vi "Connection Test.vi"() -> ()   [LabVIEW 2015]
uses:
  <vilib>/Rock Robotics/SystemInterfaces/spilib/spi_bus.ctl
  <vilib>/Platform/TimedLoop/XDataNode/timing_clust.ctl
  <vilib>/Platform/TimedLoop/XDataNode/nitl_modes.ctl
  <vilib>/Platform/TimedLoop/XDataNode/wakeup.ctl
  <vilib>/Rock Robotics/SystemInterfaces/i2clib/i2c_bus.ctl
  navX Library v3/navX Registry Cache/_TypeDefs/DeviceRegistryTypeDef.ctl
  navX Library v3/navX/navX.lvclass/navX.ctl
  navX Library v3/navX - Interface/navX - Interface.lvclass/navX - Interface.ctl
  navX Library v3/navX/_Open/OpenSPI.vi
  navX Library v3/navX - Interface/Notifications/Send Notification.vi
  <vilib>/platform/TimedLoop/XDataNode/XDataNode.xnode
  navX Library v3/navX - Interface/navX - Interface.lvclass
  navX Library v3/navX/navX.lvclass
  <vilib>/Platform/TimedLoop/XDataNode/XDNodeRunTimeDep.lvlib
  navX Library v3/navX Registry Cache/navX Registry Cache.lvclass
panel:
  out "Timestamp":u32
  in  "Update Rate (4Hz-100Hz)":u8=4 min=4 max=100 step=1
  in  "Update Button":bool
  out "YPRHfH":T1
  in  "stop":bool
  out "Iteration Duration":i64
  out "Finished Late? [i-1]":bool
  out "Registry":u8[][](array[numeric])
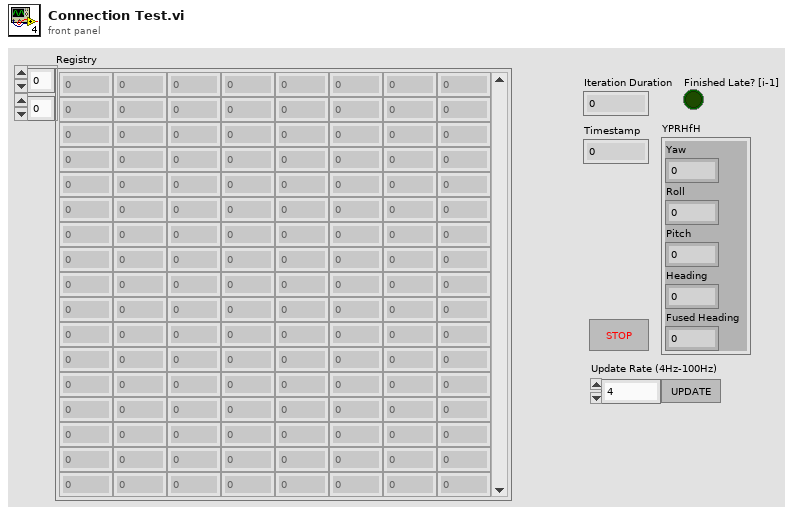
[diagram p1: front panel]
types:
  T1 = cluster{"Yaw":dbl, "Roll":dbl, "Pitch":dbl, "Heading":dbl, "Fused Heading":dbl}
  T2 = typedef "i2c_bus.ctl" = enum16{"I2C On-Board", "I2C MXP", "Invalid"}
  T3 = typedef "spi_bus.ctl" = enum16{"SPI On-Board, CS0", "SPI On-Board, CS1", "SPI On-Board, CS2", "SPI On-Board, CS3", "SPI MXP", "Invalid"}
  T4 = typedef "XDNodeRunTimeDep.lvlib/timing_clust.ctl" = cluster{"Expected End [f-1]":u64, "Actual End [f-1]":u64, "Finished Late? [f-1]":bool, "Expected End [i-1]":u64, "Actual End [i-1]":u64, "Finished Late? [i-1]":bool, "Expected Start [i]":u64, "Actual Start [i]":u64, "Expected Start [f]":u64, "Actual Start [f]":u64, "Source Name":string, "Structure Name":string, "Period":i64, "Deadline":i64, "Offset":i64, "Start":i64, "Priority":i32, "Timeout":i32, "Mode":T5, "Wakeup Reason":T6, "Error":errorcluster, "Source Type":string, "Secondary Source Type":string, "Global End Time":u64, "Global Start Time":u64, "Frame Duration":u64, "Iteration Duration":u64, "Assigned CPU":i32, "I/O Scan Engine Mode":u32}
  T5 = typedef "XDNodeRunTimeDep.lvlib/nitl_modes.ctl" = enum32{"No Change", "Process missed periods, maintain original phase", "Discard missed periods, maintain original phase", "Process missed periods, ignore original phase", "Discard missed periods, ignore original phase"}
  T6 = typedef "XDNodeRunTimeDep.lvlib/wakeup.ctl" = enum32{"Normal", "Aborted", "Asynchronous wakeup", "Timing source error", "Timed loop error", "Timeout"}
  T7 = typedef "navX Library v3.lvlib/navX Registry Cache.lvclass/DeviceRegistryTypeDef.ctl" = u8
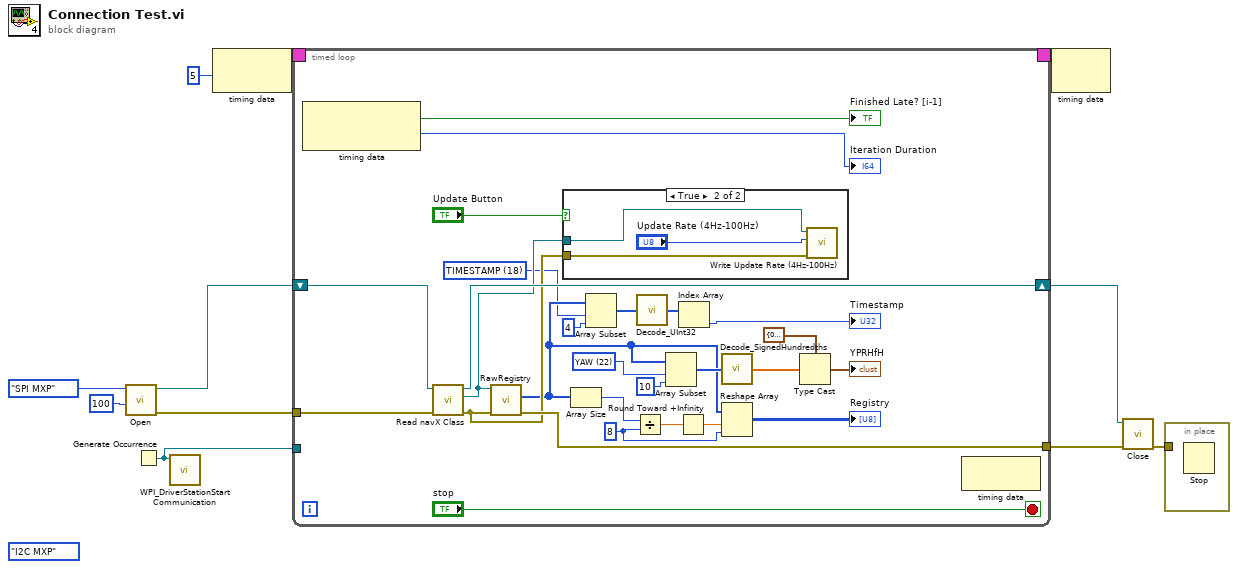
[diagram p0: block diagram]
diagram:
  (unwired) i2c_bus."I2C MXP" ("I2C Bus")
  n1 = call-poly "Open.vi"("Update Rate (4Hz-100Hz)"=u8 100, "SPI Bus"=spi_bus."SPI MXP") -> ("error out"=w8:errorcluster, "navX out"=w7:refnum<class "navX.lvclass">)  [unwired: 8 in]
  n2 = Generate Occurrence() -> (w2:refnum<k4>)
  n3 = call <vilib>:"WPI_DriverStationStart Communication.vi"("occurrence"=w2) -> ()  [unwired: 11 in]
  n4 = node-c288(i64 5 ("Period")) -> (w10:T4)
  n5 = timed-loop {
    timing: w10 -> [_]
    timing-out: [_] -> w9
    tunnel: w8 -> [w27]
    tunnel: [w37] -> w6
    tunnel: w2 -> [_]
    shift-right: [w36] -> w5
    shift-left: w7 -> [w38]
    stop <- "stop" stop-if-true
    w15 = T7 18 items=["WHOAMI"=0, "HW_REV"=1, "FW_VER_MAJOR"=2, "FW_VER_MINOR"=3, "UPDATE_RATE_HZ"=4, "ACCEL_FSR_G"=5, "GYRO_FSR_DPS"=6, "OP_STATUS"=8, "CAL_STATUS"=9, "SELFTEST_STATUS"=10, "CAPABILITY_FLAGS_L"=11, "CAPABILITY_FLAGS_H"=12, "SENSOR_STATUS"=16, "TIMESTAMP"=18, "YAW"=22, "ROLL"=24, "PITCH"=26, "HEADING"=28, "FUSED_HEADING"=30, "ALTITUDE_I"=32, "ALTITUDE_D"=34, "LINERA_ACC_X"=36, "LINERA_ACC_Y"=38, "LINERA_ACC_Z"=40, "QUAT_W"=42, "QUAT_X"=44, "QUAT_Y"=46, "QUAT_Z"=48, "MPU_TEMP_C"=50, "GYRO_X"=52, "GYRO_Y"=54, "GYRO_Z"=56, "ACC_X"=58, "ACC_Y"=60, "ACC_Z"=62, "MAG_X"=64, "MAG_Y"=66, "MAG_Z"=68, "PRESSURE_I"=70, "PRESSURE_D"=72, "PRESSURE_TEMP"=74, "YAW_OFFSET"=76, "QUAT_OFFSET_W"=78, "QUAT_OFFSET_X"=80, "QUAT_OFFSET_Y"=82, "QUAT_OFFSET_Z"=84, "INTEGRATION_CONTROL"=86, "VELOCITY_X"=88, "VELOCITY_Y"=92, "VELOCITY_Z"=96, "DISPLACMENT_X"=100, "DISPLACMENT_Y"=104, "DISPLACEMENT_Z"=108] ("Device Register")
    w26 = 8 ("dimension size")
    w32 = T7 22 items=["WHOAMI"=0, "HW_REV"=1, "FW_VER_MAJOR"=2, "FW_VER_MINOR"=3, "UPDATE_RATE_HZ"=4, "ACCEL_FSR_G"=5, "GYRO_FSR_DPS"=6, "OP_STATUS"=8, "CAL_STATUS"=9, "SELFTEST_STATUS"=10, "CAPABILITY_FLAGS_L"=11, "CAPABILITY_FLAGS_H"=12, "SENSOR_STATUS"=16, "TIMESTAMP"=18, "YAW"=22, "ROLL"=24, "PITCH"=26, "HEADING"=28, "FUSED_HEADING"=30, "ALTITUDE_I"=32, "ALTITUDE_D"=34, "LINERA_ACC_X"=36, "LINERA_ACC_Y"=38, "LINERA_ACC_Z"=40, "QUAT_W"=42, "QUAT_X"=44, "QUAT_Y"=46, "QUAT_Z"=48, "MPU_TEMP_C"=50, "GYRO_X"=52, "GYRO_Y"=54, "GYRO_Z"=56, "ACC_X"=58, "ACC_Y"=60, "ACC_Z"=62, "MAG_X"=64, "MAG_Y"=66, "MAG_Z"=68, "PRESSURE_I"=70, "PRESSURE_D"=72, "PRESSURE_TEMP"=74, "YAW_OFFSET"=76, "QUAT_OFFSET_W"=78, "QUAT_OFFSET_X"=80, "QUAT_OFFSET_Y"=82, "QUAT_OFFSET_Z"=84, "INTEGRATION_CONTROL"=86, "VELOCITY_X"=88, "VELOCITY_Y"=92, "VELOCITY_Z"=96, "DISPLACMENT_X"=100, "DISPLACMENT_Y"=104, "DISPLACEMENT_Z"=108] ("Device Register")
    n6 = node-c288() -> (→"Finished Late? [i-1]":bool, →"Iteration Duration":i64)  [unwired: 1 in]
    n7 = call "Read navX Class.vi"("error in (no error)"=w27, "navX in"=w38) -> ("error out"=w19:errorcluster, "navX Library v3.lvlib:navX - Base.lvclass"=w20:refnum<class "navX - Interface.lvclass">, "navX out"=w36:refnum<class "navX.lvclass">)  [unwired: 7 in]
    n8 = call "RawRegistry.vi"("error in (no error)"=w19, "navX - Base in"=w20) -> ("error out"=w37:errorcluster, "Registry Cache out"=w16:u8[])  [unwired: 7 in, 1 out]
    n9 = case shown="True" "Update Button" {
      tunnel: w20 -> [_ w41]
      tunnel: w19 -> [_ w39]
      frame False {
      }
      frame True {
        n10 = call "Write Update Rate (4Hz-100Hz).vi"("error in (no error)"=w39, "Update Rate (4Hz-100Hz)"="Update Rate (4Hz-100Hz)", "navX - Base in"=w41) -> ()  [unwired: 7 in, 2 out]
      }
    }
    n11 = Array Size(array=w16) -> (size(s)=w23:i32)
    n12 = Array Subset(array=w16, index=w15, length=4) -> (w14:u8[])
    n13 = Divide(x=w23, y=w26) -> (x/y=w24:dbl)
    n14 = call "Decode_UInt32.vi"("Little Endian"=w14) -> ("UInt32"=w13:u32[])
    n15 = Array Subset(array=w16, index=w32, length=10) -> (w17:u8[])
    n16 = Round Toward +Infinity(x=w24) -> (ceil(x): smallest int >= x=w25:dbl)
    n17 = Index Array(array=w13) -> (element=→"Timestamp":u32)  [unwired: 1 in]
    n18 = call "Decode_SignedHundredths.vi"("Little Endian"=w17) -> ("Signed Hundredths (0.00)"=w29:dbl[])
    n19 = Reshape Array(w16, w25, w26) -> (→"Registry":u8[][])
    n20 = Type Cast(type=T1 {"Yaw"=0.0, "Roll"=0.0, "Pitch"=0.0, "Heading"=0.0, "Fused Heading"=0.0}, x=w29) -> (*(type *) &x=→"YPRHfH":T1)
    n21 = node-c288() -> ()  [unwired: 1 in, 1 out]
  }
  n22 = node-c288(w9) -> ()  [unwired: 1 out]
  n23 = call "Close.vi"("error in (no error)"=w6, "navX in"=w5) -> ("error out"=w1:errorcluster)  [unwired: 9 in]
  n24 = in-place {
    in-place-border: w1 -> [_]
    n25 = Stop() -> ()  [unwired: 1 in]
  }
